vi "AdjustBounds.vi"(6 "T minimum":dbl, 7 "T maximum":dbl, 9 "DAQ3 Plots (cut)":refnum<vi>, 10 "DAQ2 Plots (cut)":refnum<vi>, 11 "DAQ3 Plots (cut)":refnum<vi>) -> ()   [LabVIEW 2013]
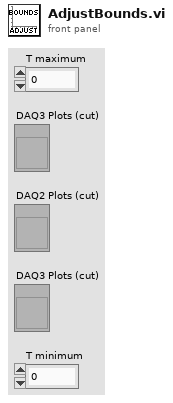
[diagram p1: front panel]
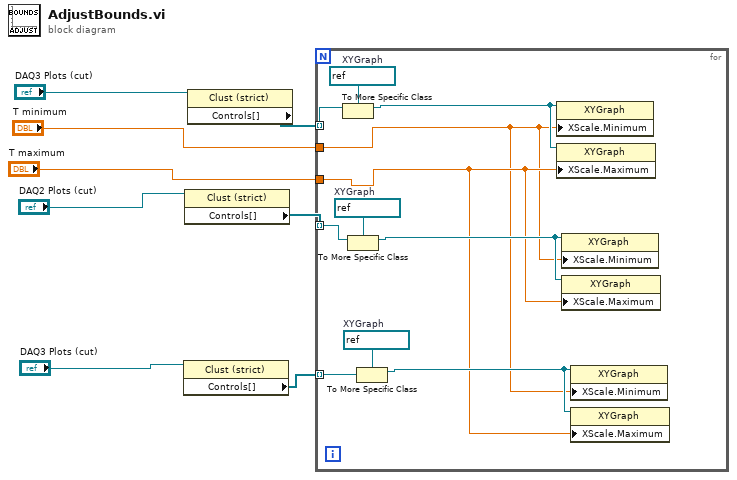
[diagram p0: block diagram]
diagram:
  n1 = property class="Clust (strict)"(reference="DAQ3 Plots (cut)") -> ("Controls[]"=w6:refnum<vi>[])  [unwired: 1 in, 2 out]
  n2 = property class="Clust (strict)"(reference="DAQ2 Plots (cut)") -> ("Controls[]"=w4:refnum<vi>[])  [unwired: 1 in, 2 out]
  n3 = property class="Clust (strict)"(reference="DAQ3 Plots (cut)") -> ("Controls[]"=w1:refnum<vi>[])  [unwired: 1 in, 2 out]
  n4 = for {
    tunnel: w1 -> [w18] mode=indexing
    tunnel: w4 -> [w14] mode=indexing
    tunnel: w6 -> [w11] mode=indexing
    tunnel: "T maximum" -> [w10]
    tunnel: "T minimum" -> [w9]
    w13 = refnum<vi> refnum  # XYGraph
    w16 = refnum<vi> refnum  # XYGraph
    w19 = refnum<vi> refnum  # XYGraph
    n5 = To More Specific Class(target class=w19, reference=w18) -> (specific class reference=w17:refnum<vi>)  [unwired: 1 in, 1 out]
    n6 = To More Specific Class(target class=w16, reference=w14) -> (specific class reference=w15:refnum<vi>)  [unwired: 1 in, 1 out]
    n7 = To More Specific Class(target class=w13, reference=w11) -> (specific class reference=w12:refnum<vi>)  [unwired: 1 in, 1 out]
    n8 = property class="XYGraph"(reference=w17, "XScale.Minimum"=w9) -> ()  [unwired: 1 in, 2 out]
    n9 = property class="XYGraph"(reference=w17, "XScale.Maximum"=w10) -> ()  [unwired: 1 in, 2 out]
    n10 = property class="XYGraph"(reference=w15, "XScale.Minimum"=w9) -> ()  [unwired: 1 in, 2 out]
    n11 = property class="XYGraph"(reference=w15, "XScale.Maximum"=w10) -> ()  [unwired: 1 in, 2 out]
    n12 = property class="XYGraph"(reference=w12, "XScale.Minimum"=w9) -> ()  [unwired: 1 in, 2 out]
    n13 = property class="XYGraph"(reference=w12, "XScale.Maximum"=w10) -> ()  [unwired: 1 in, 2 out]
  }
